vi "Log.vi"(8 "error in":errorcluster, 9 "Meta Data":string[](array[string]), 10 "String Data":string[](array[string]), 11 "File Logger Interface in":refnum<class "File Type Interface.lvclass">) -> (0 "error out":errorcluster, 3 "File Logger Interface out":refnum<class "File Type Interface.lvclass">)   [LabVIEW 2020, in "File Type Interface.lvclass"]
uses:
  File Type Interface.lvclass
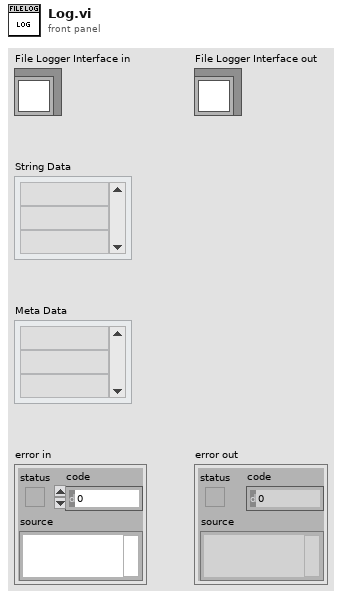
[diagram p1: front panel]
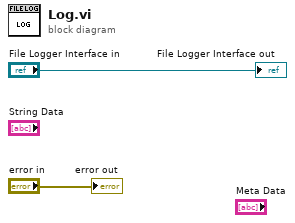
[diagram p0: block diagram]
diagram:
  "error out" <- "error in"
  "File Logger Interface out" <- "File Logger Interface in"
